vi "QE Reset.vi"   [LabVIEW 2013, in "LVH-LINX.lvlib"]
doc: "Set counter value(s) to 0 for the specified quadrature encoder channel(s)."
uses:
  LVH-LINX.lvlib
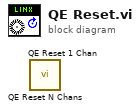
[diagram p0: block diagram]
diagram:
  n1 = call "QE Reset N Chans.vi"() -> ()  [unwired: 10 in, 2 out]
  n2 = call "QE Reset 1 Chan.vi"() -> ()  [unwired: 10 in, 2 out]
